vi "Check Labels.vi"(0 "Metric in":refnum<class "Metric.lvclass">, 12 "Labels":map{string, string}(c390)) -> (4 "Samples":map{string, refnum<class "Sample.lvclass">}(c390), 6 "Valid Labels":bool, 8 "Label Values":string[](array[string]))   [LabVIEW 2020, in "Metrics.lvlib" / "Metric.lvclass"]
uses:
  Metric.lvclass
  sample/Sample.lvclass
  Metric.lvclass/Metric.ctl
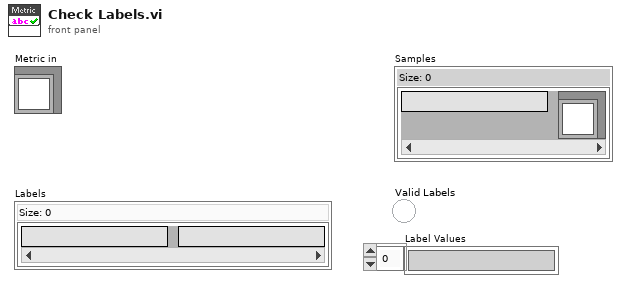
[diagram p1: front panel]
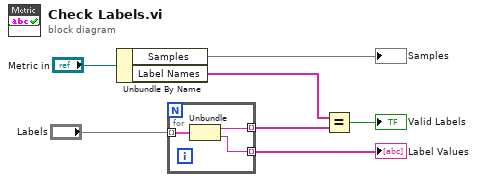
[diagram p0: block diagram]
diagram:
  n1 = Unbundle By Name("Metric in") -> ("Samples"=→"Samples":map{string, refnum<class "Sample.lvclass">}, "Label Names"=w4:string[])
  n2 = for {
    tunnel: "Labels" -> [w10] mode=indexing
    tunnel: [w9] -> w1 mode=indexing
    tunnel: [w8] -> w7 mode=indexing
    n3 = Unbundle(w10) -> ("labelname"=w9:string, "labelvalue"=w8:string)
  }
  "Label Values" <- w7
  n4 = Equal?(x=w4, y=w1) -> (x = y?=→"Valid Labels":bool)
